vi "Write Python version.vi"(8 "error in (no error)":errorcluster, 10 "Python version":string="3.6", 11 "User.Python in":refnum<class "User.Python.lvclass">) -> (0 "error out":errorcluster, 3 "User.Python out":refnum<class "User.Python.lvclass">)   [LabVIEW 2019, in "User.Python.lvclass"]
doc: "Vesion must match the Python version you have installed and wish to call. Note that the bitness must match the LabVIEW version being called.\n\nExample: To call Python 3.8.1 type 3.8"
uses:
  User.Python.lvclass
  User.Python.lvclass/User.Python.ctl
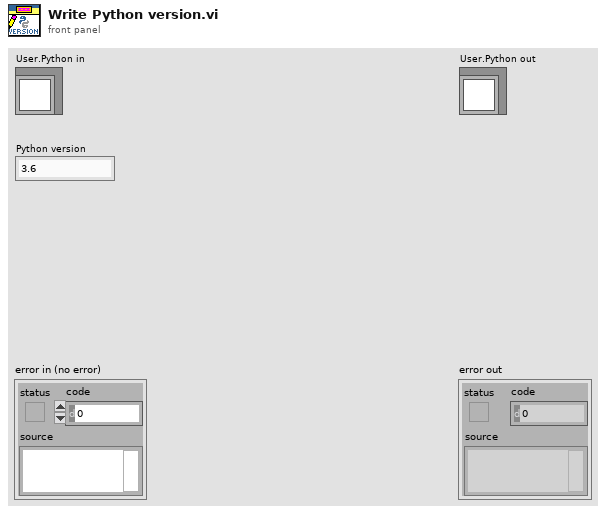
[diagram p1: front panel]
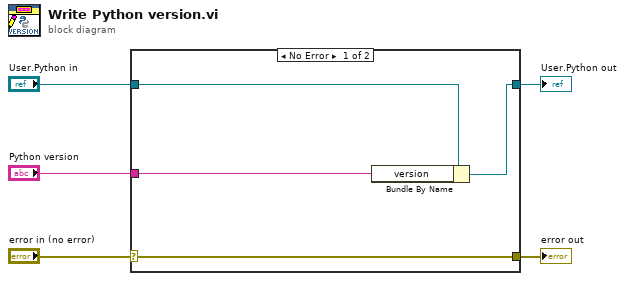
[diagram p0: block diagram]
diagram:
  n1 = case shown="No Error" "error in (no error)" {
    selector: "error in (no error)" -> [w9 w10]
    tunnel: [w9 w10] -> w4
    tunnel: [w7 w11] -> w2
    tunnel: "User.Python in" -> [w8 w11]
    tunnel: "Python version" -> [w6 _]
    frame No Error {
      n2 = Bundle By Name(cluster=w8, "version"=w6) -> (w7:refnum<class "User.Python.lvclass">)
    }
    frame Error {
    }
  }
  "error out" <- w4
  "User.Python out" <- w2
